vi "SubVI_ReadRow.vi"(11 "String":string) -> (3 "Row":dbl[](array[numeric]))   [LabVIEW 2011]
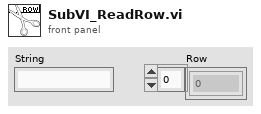
[diagram p1: front panel]
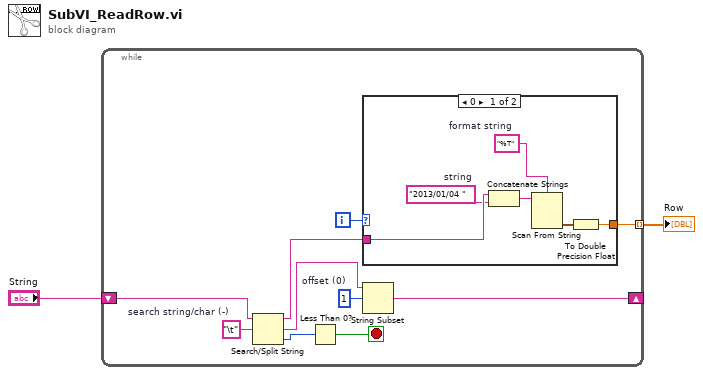
[diagram p0: block diagram]
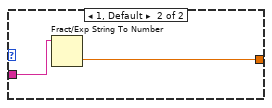
[diagram p2: hidden frame]
diagram:
  n1 = while {
    shift-right: [w6] -> _
    shift-left: "String" -> [w12]
    tunnel: [w7] -> w1 mode=indexing
    i -> [w3]
    stop <- w5 stop-if-true
    w10 = 1  # offset (0)
    w11 = "\t"  # search string/char (-)
    n2 = Search/Split String(string=w12, search string/char (-)=w11) -> (substring before match=w8:string, match + rest of string=w9:string, offset of match=w4:i32)  [unwired: 1 in]
    n3 = Less Than 0?(x=w4) -> (x < 0?=w5:bool)
    n4 = case shown="0" w3 {
      tunnel: w8 -> [w18 w20]
      tunnel: [w13 w19] -> w7
      frame 0 {
        w14 = "%T"  # format string
        w15 = "2013/01/04 "  # string
        n5 = Concatenate Strings(w18, w15) -> (w16:string)
        n6 = Scan From String(format string=w14, input string=w16) -> (output 1=w17:timestamp)  [unwired: 3 in, 3 out]
        n7 = To Double Precision Float(number=w17) -> (double precision float=w13:dbl)
      }
      frame 1, Default {
        n8 = Fract/Exp String To Number(string=w20) -> (number=w19:dbl)  [unwired: 3 in, 1 out]
      }
    }
    n9 = String Subset(string=w9, offset (0)=w10) -> (substring=w6:string)  [unwired: 1 in]
  }
  "Row" <- w1
